vi "LM model function Raman polybaseline.vi"(3 "output control":T1, 4 "data":T2, 5 "X":dbl[](array[numeric]) format="%#_8g", 6 "a":dbl[](array[numeric])) -> (0 "error out":errorcluster, 1 "f'(X,a)":dbl[][](array[numeric]), 2 "f(X,a)":dbl[](array[numeric]))   [LabVIEW 2015]
doc: "This template is the starting point for creating a model function to be passed to the Nonlinear Curve Fit.vi."
uses:
  <vilib>/gmath/NumericalOptimization/objective function data.ctl
  <vilib>/gmath/NumericalOptimization/LM_output select.ctl
  <vilib>/Utility/file.llb/Read From Spreadsheet File (DBL).vi
  <vilib>/gmath/NI_Gmath.lvlib
panel:
  # "Version 1.0\nAVM"
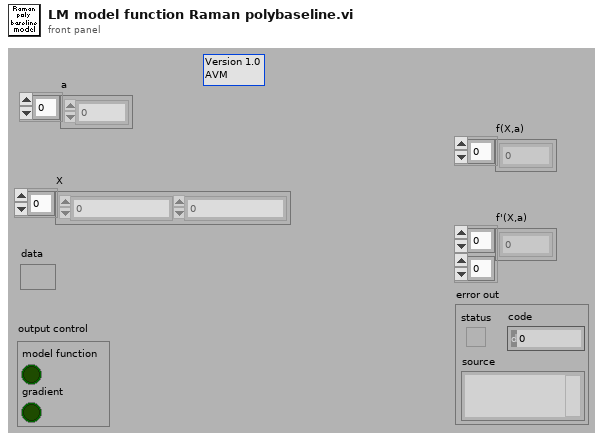
[diagram p1: front panel]
types:
  T1 = typedef "NI_Gmath.lvlib/LM_output select.ctl" = cluster{"model function":bool, "gradient":bool}
  T2 = typedef "NI_Gmath.lvlib/objective function data.ctl" = variant
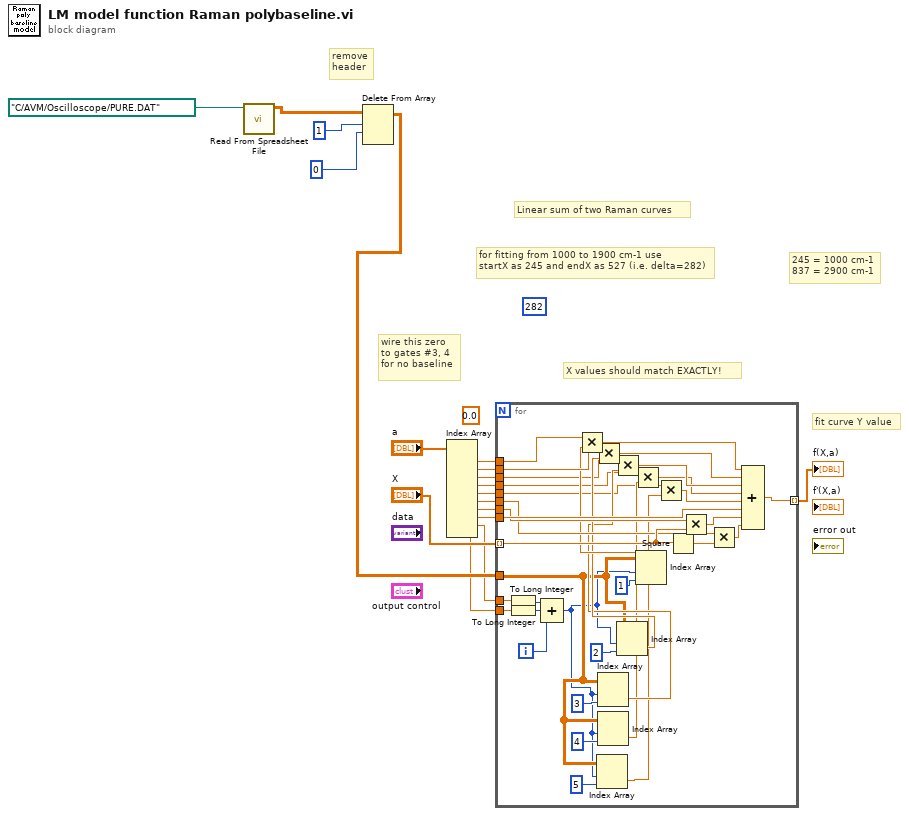
[diagram p0: block diagram]
diagram:
  (unwired) 282 ("index (row)")
  (unwired) 0.0 ("element")
  # "245 = 1000 cm-1\n837 = 2900 cm-1"
  # "for fitting from 1000 to 1900 cm-1 use\nstartX as 245 and endX as 527 (i.e. delta=282)"
  # "wire this zero\nto gates #3, 4\nfor no baseline"
  # "remove\nheader"
  # "X values should match EXACTLY!"
  # "Linear sum of two Raman curves"
  # "fit curve Y value"
  n1 = call-poly <vilib>:"Read From Spreadsheet File.vi"("file path (dialog if empty)"=path "C:/AVM/Oscilloscope/PURE.DAT") -> ("all rows"=w14:dbl[][])  [unwired: 6 in, 4 out]
  n2 = Delete From Array(array=w14, length=1 ("index (row)"), index (row)=0) -> (array with subset deleted=w9:dbl[][])  [unwired: 1 in, 1 out]
  n3 = Index Array(array="a") -> (element #1=w17:dbl, element #2=w16:dbl, element #3=w8:dbl, element #4=w7:dbl, element #5=w1:dbl, element #6=w2:dbl, element #7=w3:dbl, element #8=w4:dbl, element #9=w6:dbl, element #10=w5:dbl)  [unwired: 10 in]
  n4 = for {
    tunnel: "X" -> [w48] mode=indexing
    tunnel: w17 -> [w22]
    tunnel: w16 -> [w36]
    tunnel: [w50] -> w15 mode=indexing
    tunnel: w9 -> [w30]
    tunnel: w8 -> [w21]
    tunnel: w7 -> [w20]
    tunnel: w6 -> [w46]
    tunnel: w5 -> [w42]
    tunnel: w4 -> [w39]
    tunnel: w3 -> [w38]
    tunnel: w2 -> [w37]
    tunnel: w1 -> [w19]
    i -> [w44]
    n5 = To Long Integer(number=w46) -> (32bit integer=w45:i32)
    n6 = To Long Integer(number=w42) -> (32bit integer=w43:i32)
    n7 = Compound Arithmetic op=ADD(w45, w43, w44) -> (w29:i32)
    n8 = Index Array(array=w30, index (row)=w29, index (col)=5 ("index (row)")) -> (element=w28:dbl)
    n9 = Index Array(array=w30, index (row)=w29, index (col)=3 ("index (row)")) -> (element=w33:dbl)
    n10 = Index Array(array=w30, index (row)=w29, index (col)=4 ("index (row)")) -> (element=w32:dbl)
    n11 = Multiply(x=w21, y=w33) -> (x*y=w25:dbl)
    n12 = Index Array(array=w30, index (row)=w29, index (col)=2 ("index (row)")) -> (element=w34:dbl)
    n13 = Multiply(x=w36, y=w34) -> (x*y=w26:dbl)
    n14 = Multiply(x=w20, y=w32) -> (x*y=w24:dbl)
    n15 = Index Array(array=w30, index (row)=w29, index (col)=1 ("index (row)")) -> (element=w35:dbl)
    n16 = Multiply(x=w22, y=w35) -> (x*y=w27:dbl)
    n17 = Multiply(x=w19, y=w28) -> (x*y=w23:dbl)
    n18 = Square(x=w48) -> (x^2=w47:dbl)
    n19 = Multiply(x=w38, y=w48) -> (x*y=w41:dbl)
    n20 = Multiply(x=w37, y=w47) -> (x*y=w40:dbl)
    n21 = Compound Arithmetic op=ADD(w27, w26, w25, w24, w23, w39, w41, w40) -> (w50:dbl)
  }
  "f(X,a)" <- w15
